vi "populate tree.vi"(6 "Tree Refnum":refnum<vi>, 8 "error in (no error)":errorcluster, 10 "Root":path) -> (0 "error out":errorcluster)   [LabVIEW 2020]
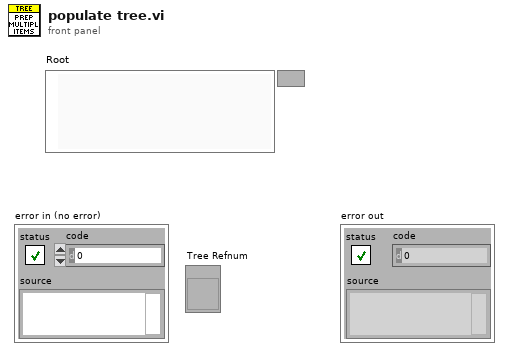
[diagram p1: front panel]
types:
  T1 = cluster{"Left Cell String":string, "Child Text":string[], "Child Tag":string, "Item Indent":i32, "Child Only?":bool, "Glyph Index":i32}[]
  T2 = cluster{"Left Cell String":string, "Child Text":string[], "Child Tag":string, "Item Indent":i32, "Child Only?":bool, "Glyph Index":i32}
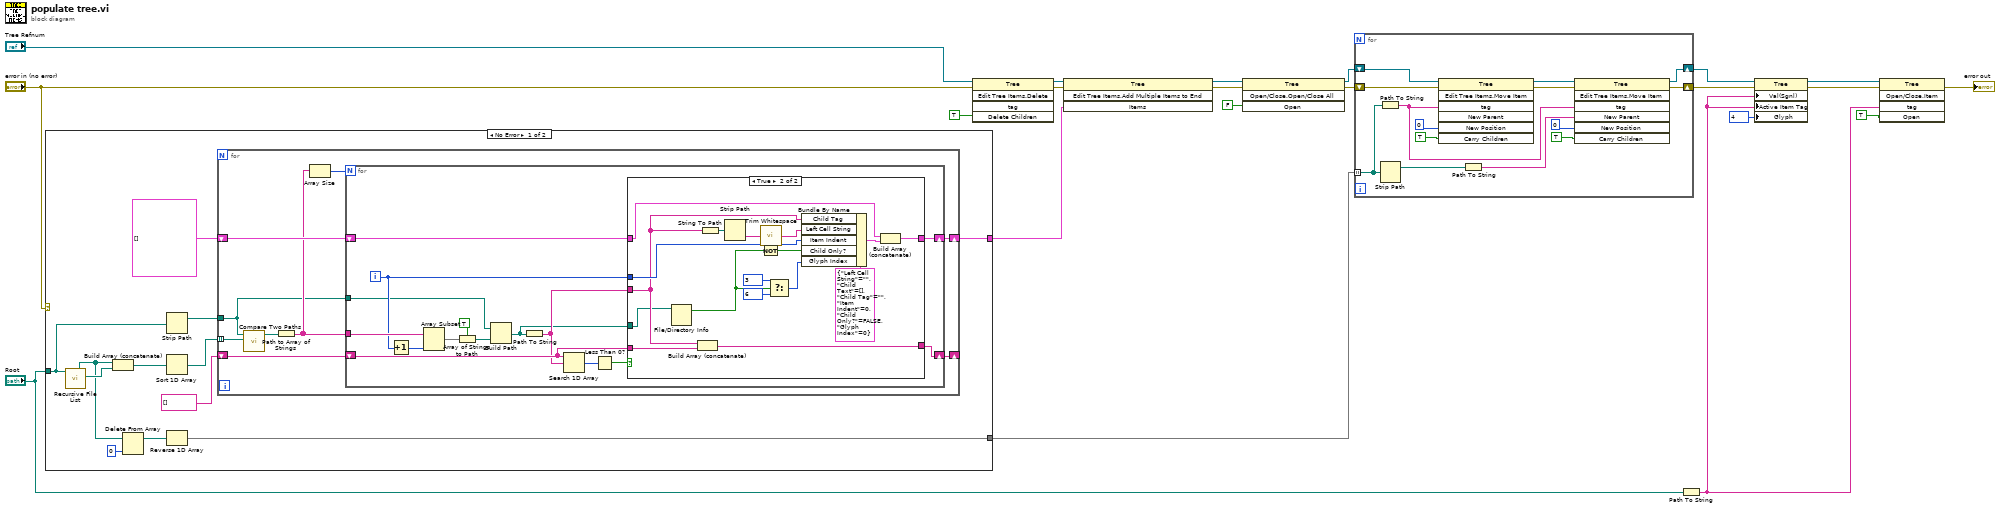
[diagram p0: block diagram]
diagram:
  n1 = case shown="No Error" "error in (no error)" {
    tunnel: [w30 _] -> w18
    tunnel: "Root" -> [w27 _]
    tunnel: [w22 _] -> w9
    frame No Error {
      n2 = call <vilib>:"Recursive File List.vi"("Folder Path"=w27) -> ("All Files in Dir"=w29:path[], "All Folders"=w25:path[])  [unwired: 2 in, 7 out]
      n3 = Build Array (concatenate)(w25, w29) -> (w28:path[])
      n4 = Delete From Array(array=w25, index=0) -> (array with subset deleted=w24:path[])  [unwired: 1 in, 1 out]
      n5 = Strip Path(path=w27) -> (stripped path=w26:path)  [unwired: 1 out]
      n6 = Sort 1D Array(array=w28) -> (sorted array=w31:path[])
      n7 = Reverse 1D Array(array=w24) -> (reversed array=w22:path[])
      n8 = for {
        tunnel: w31 -> [w35] mode=indexing
        shift-right: [w37] -> w30
        shift-left: T1 [] -> [w42]
        shift-right: [w39] -> _
        shift-left: string[] [] -> [w41]
        tunnel: w26 -> [w34]
        n9 = call <vilib>:"Compare Two Paths.vi"("Path 2"=w35, "Path 1"=w34) -> ("Relative Path from 1 to 2"=w36:path)  [unwired: 1 in, 8 out]
        n10 = Path to Array of Strings(0:w36) -> (2:w40:string[])  [unwired: 1 out]
        n11 = Array Size(array=w40) -> (size(s)=w38:i32)
        n12 = for {
          N: w38 -> [_]
          tunnel: w40 -> [w54]
          shift-right: [w52] -> w37
          shift-left: w42 -> [w56]
          shift-right: [w53] -> w39
          shift-left: w41 -> [w55]
          tunnel: w34 -> [w47]
          i -> [w51]
          n13 = Increment(x=w51) -> (x+1=w43:i32)
          n14 = Array Subset(array=w54, length=w43) -> (w49:string[])  [unwired: 1 in]
          n15 = Array of Strings to Path(0:w49, 1:TRUE ("relative")) -> (2:w46:path)
          n16 = Build Path(base path=w47, name or relative path=w46) -> (appended path=w44:path)
          n17 = Path To String(path=w44) -> (string=w45:string)
          n18 = Search 1D Array(1D array=w55, element=w45) -> (index of element=w57:i32)  [unwired: 1 out]
          n19 = Less Than 0?(x=w57) -> (x < 0?=w50:bool)
          n20 = case shown="True" w50 {
            tunnel: w56 -> [w58 w75]
            tunnel: w55 -> [w59 w73]
            tunnel: w45 -> [_ w71]
            tunnel: [w59 w72] -> w53
            tunnel: w51 -> [_ w76]
            tunnel: [w58 w74] -> w52
            tunnel: w44 -> [_ w63]
            frame False {
            }
            frame True {
              n21 = File/Directory Info(path=w63) -> (directory=w62:bool)  [unwired: 1 in, 6 out]
              n22 = Build Array (concatenate)(w71, w73) -> (w72:string[])
              n23 = String To Path(string=w71) -> (path=w69:path)
              n24 = Strip Path(path=w69) -> (name=w68:string)  [unwired: 1 out]
              n25 = Not(x=w62) -> (.not. x?=w65:bool)
              n26 = call <vilib>:"Trim Whitespace.vi"("string"=w68) -> ("trimmed string"=w67:string)  [unwired: 1 in]
              n27 = Select(t=3, s=w62, f=6) -> (s? t:f=w66:i32)
              n28 = Bundle By Name(cluster=T2 {"Left Cell String"="", "Child Text"=[], "Child Tag"="", "Item Indent"=0, "Child Only?"=FALSE, "Glyph Index"=0} ("Item"), "Child Tag"=w71, "Left Cell String"=w67, "Item Indent"=w76, "Child Only?"=w65, "Glyph Index"=w66) -> (w70:T2)
              n29 = Build Array (concatenate)(w75, w70) -> (w74:T1)
            }
          }
        }
      }
    }
    frame Error {
    }
  }
  n30 = invoke on="Invoke Node" class="Tree" method="Edit Tree Items.Delete"(reference="Tree Refnum", error in="error in (no error)", "Delete Children"=TRUE ("Delete Children?")) -> (reference out=w20:refnum<vi>, error out=w19:errorcluster)  [unwired: 2 in, 3 out]
  n31 = invoke on="Invoke Node" class="Tree" method="Edit Tree Items.Add Multiple Items to End"(reference=w20, error in=w19, "Items"=w18) -> (reference out=w16:refnum<vi>, error out=w15:errorcluster)  [unwired: 1 in, 2 out]
  n32 = invoke on="Invoke Node" class="Tree" method="Open/Close.Open/Close All"(reference=w16, error in=w15, "Open"=FALSE ("Open?")) -> (reference out=w13:refnum<vi>, error out=w12:errorcluster)  [unwired: 1 in, 2 out]
  n33 = for {
    shift-right: [w78] -> w11
    shift-left: w13 -> [w90]
    shift-right: [w77] -> w10
    shift-left: w12 -> [w89]
    tunnel: w9 -> [w84] mode=indexing
    n34 = Path To String(path=w84) -> (string=w79:string)
    n35 = Strip Path(path=w84) -> (stripped path=w83:path)  [unwired: 1 out]
    n36 = invoke on="Invoke Node" class="Tree" method="Edit Tree Items.Move Item"(reference=w90, error in=w89, "tag"=w79, "New Position"=0, "Carry Children"=TRUE ("Carry Children?")) -> (reference out=w86:refnum<vi>, error out=w85:errorcluster)  [unwired: 2 in, 5 out]
    n37 = Path To String(path=w83) -> (string=w82:string)
    n38 = invoke on="Invoke Node" class="Tree" method="Edit Tree Items.Move Item"(reference=w86, error in=w85, "tag"=w79, "New Parent"=w82, "New Position"=0, "Carry Children"=TRUE ("Carry Children?")) -> (reference out=w78:refnum<vi>, error out=w77:errorcluster)  [unwired: 1 in, 5 out]
  }
  n39 = Path To String(path="Root") -> (string=w6:string)
  n40 = property class="Tree"(reference=w11, error in=w10, "Val(Sgnl)"=w6, "Active Item Tag"=w6, "Glyph"=4) -> (reference out=w8:refnum<vi>, error out=w7:errorcluster)
  n41 = invoke on="Invoke Node" class="Tree" method="Open/Close.Item"(reference=w8, error in=w7, "tag"=w6, "Open"=TRUE ("Open?")) -> (error out=→"error out":errorcluster)  [unwired: 1 in, 4 out]
